vi "Remove Blank Columns (2D String Array).vi"(4 "Array In":string[][](array[string])) -> (18 "Array Out":string[][](array[string]))   [LabVIEW 2013]
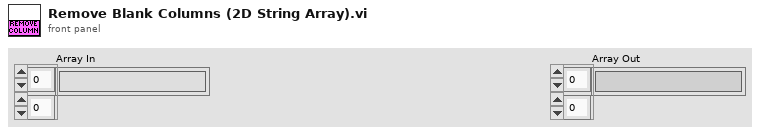
[diagram p1: front panel]
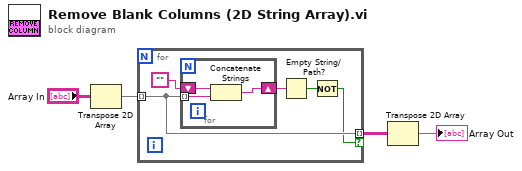
[diagram p0: block diagram]
diagram:
  n1 = Transpose 2D Array(2D array="Array In") -> (transposed array=w3:string[][])
  n2 = for {
    tunnel: w3 -> [w8] mode=indexing
    tunnel: [w8] -> w2 mode=indexing if=w5
    n3 = for {
      tunnel: w8 -> [w11] mode=indexing
      shift-right: [w10] -> w7
      shift-left: "" -> [w12]
      n4 = Concatenate Strings(w12, w11) -> (w10:string)
    }
    n5 = Empty String/Path?(string/path=w7) -> (empty?=w6:bool)
    n6 = Not(x=w6) -> (.not. x?=w5:bool)
  }
  n7 = Transpose 2D Array(2D array=w2) -> (transposed array=→"Array Out":string[][])
